vi "CloseSession.vi"   [LabVIEW 2018]
uses:
  <vilib>/Plasmionique/MB Master/MB_Master/MB_Master.lvclass
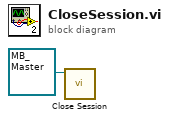
[diagram p0: block diagram]
diagram:
  n1 = call-dynamic "Close Session.vi"("MB session in"=refnum<class "MB_Master.lvclass"> refnum) -> ()  [unwired: 10 in, 1 out]
